vi "Distributor - SEND - Triggered Event.vi"(8 "error in (no error)":errorcluster, 10 "Actor_Interface.lvlib:Interface_Class.lvclass":refnum<class "Abstraction_Interface_Class.lvclass">, 11 "Parent_Class in":refnum<class "Message_Distributor_Class.lvclass">) -> (0 "error out":errorcluster, 3 "Parent_Class out":refnum<class "Message_Distributor_Class.lvclass">)   [LabVIEW 2023, in "Actor_Message_Distributor.lvlib" / "Message_Distributor_Class.lvclass"]
uses:
  Message_Distributor_Class.lvclass
  Abstraction_Interface_Class/Abstraction_Interface_Class.lvclass
  Message_Distributor_Class.lvclass/Message_Distributor_Class.ctl
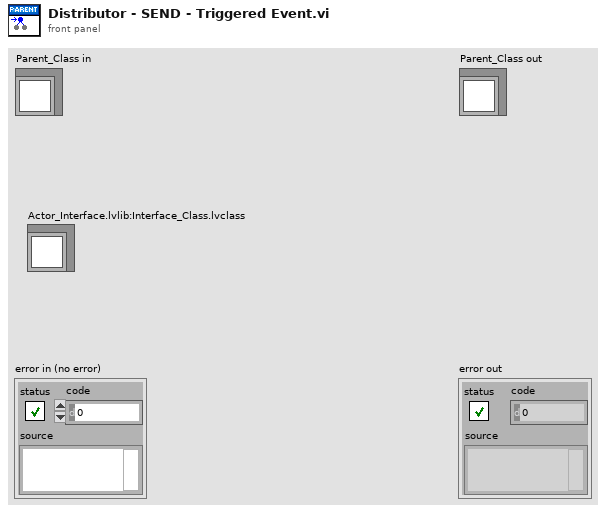
[diagram p1: front panel]
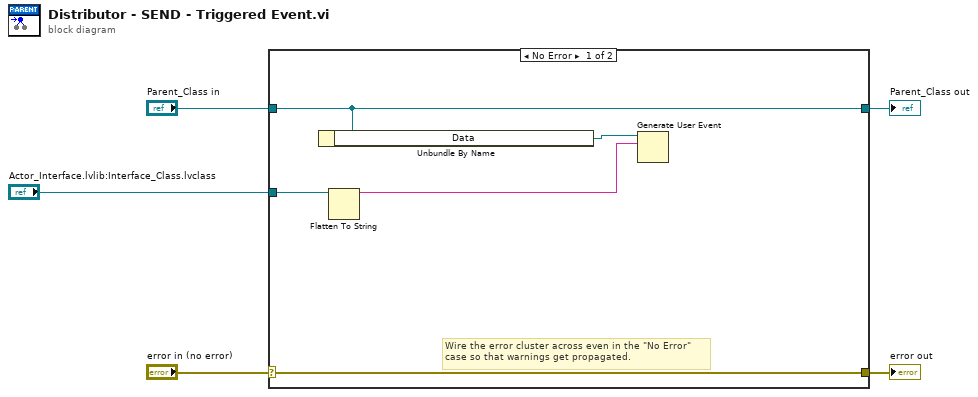
[diagram p0: block diagram]
diagram:
  n1 = case shown="No Error" "error in (no error)" {
    selector: "error in (no error)" -> [w10 w12]
    tunnel: [w10 w12] -> w4
    tunnel: [w8 w11] -> w2
    tunnel: "Parent_Class in" -> [w8 w11]
    tunnel: "Actor_Interface.lvlib:Interface_Class.lvclass" -> [w9 _]
    frame No Error {
      # "Wire the error cluster across even in the \"No Error\"\ncase so that warnings get propagated."
      n2 = Unbundle By Name(w8) -> ("Data"=w7:refnum<user-event>)
      n3 = Flatten To String(anything=w9) -> (data string=w6:string)  [unwired: 3 in, 2 out]
      n4 = Generate User Event(user event=w7, event data cluster=w6) -> ()  [unwired: 2 in, 2 out]
    }
    frame Error {
    }
  }
  "error out" <- w4
  "Parent_Class out" <- w2
